vi "GT Get Crd Vel.vi"(8 "error in (no error)":errorcluster caption="错误输入（无错误）", 9 "pSynVel":dbl, 10 "crd":i16, 11 "cardNum":i16) -> (0 "error out":errorcluster caption="错误输出", 1 "pSynVel out":dbl, 3 "function return":i16)   [LabVIEW 2014, in "gts.lvlib"]
doc: "GT_API GT_GetCrdVel(short cardNum,short crd,double *pSynVel);"
uses:
  gts.lvlib
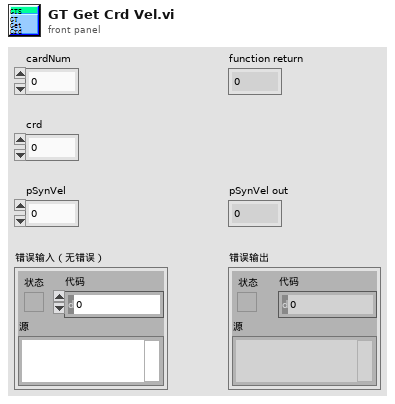
[diagram p1: front panel]
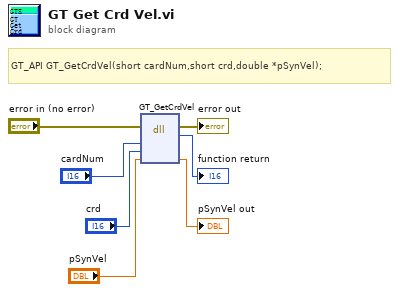
[diagram p0: block diagram]
diagram:
  # "GT_API GT_GetCrdVel(short cardNum,short crd,double *pSynVel);"
  n1 = dll-call lib="PTH2habs D固高科技资料GTS控制卡GTS卡18年上半年资料dllVC32bit\nmulti_cardgts.*" fn="GT_GetCrdVel"(error in="error in (no error)", "cardNum"="cardNum", "crd"="crd", "pSynVel"="pSynVel") -> (error out=→"error out":errorcluster, →"function return":i16, "pSynVel"=→"pSynVel out":dbl)  [unwired: 4 in, 1 out]
